vi "Marker Draw and Commands Loop.vi"(9 "Command":T1={"cmd"=enum."type", "Type"=enum."vert", "Coords"={"Horizontal"=0, "Vertical"=0}, "text"=""}, 10 "SPECTRUM":refnum<vi>, 11 "Data in":T7={"PLACEHOLDER"="", "Graph Selection"={"Options"={"Color"=16723218, "pen"={"Width"=2, "Style"=enum."Solid"}, "font"={"Font Name"="Arial", "Size"=14, "Strikeout?"=FALSE, "Italic?"=FALSE, "Underline?"=FALSE, "Outline?"=FALSE, "Shadow?"=FALSE, "Bold?"=FALSE, "FontColor"=6908265}, "caption"="Click to set a point marker"}, "Markers"={"Type"=enum."point", "X"=0.0, "Y"=0.0, "X2"=0.0, "Y2"=0.0, "Text"=""}, "state"={"cmd"=enum."click", "Type"=enum."horiz range", "Coords"={"Horizontal"=0, "Vertical"=0}, "Active Tool"=0, "mode"=enum."none"}}, "Refs"={"Source VI"=refnum, "Graph"=refnum}, "Source Ctrl Label"="", "Channel Peak"=0.0, "Mouse Init Pos"={"Horizontal"=0, "Vertical"=0, "Scrolling"=0}, "Mouse Current Pos"={"Horizontal"=0, "Vertical"=0, "Scrolling"=0}}) -> (3 "Data out":T7={"PLACEHOLDER"="", "Graph Selection"={"Options"={"Color"=16723218, "pen"={"Width"=2, "Style"=enum."Solid"}, "font"={"Font Name"="Arial", "Size"=14, "Strikeout?"=FALSE, "Italic?"=FALSE, "Underline?"=FALSE, "Outline?"=FALSE, "Shadow?"=FALSE, "Bold?"=FALSE, "FontColor"=6908265}, "caption"="Click to set a point marker"}, "Markers"={"Type"=enum."point", "X"=0.0, "Y"=0.0, "X2"=0.0, "Y2"=0.0, "Text"=""}, "state"={"cmd"=enum."click", "Type"=enum."horiz range", "Coords"={"Horizontal"=0, "Vertical"=0}, "Active Tool"=0, "mode"=enum."none"}}, "Refs"={"Source VI"=refnum, "Graph"=refnum}, "Source Ctrl Label"="", "Channel Peak"=0.0, "Mouse Init Pos"={"Horizontal"=0, "Vertical"=0, "Scrolling"=0}, "Mouse Current Pos"={"Horizontal"=0, "Vertical"=0, "Scrolling"=0}})   [LabVIEW 2019]
doc: "This draw loop is the command processor thread and redraw thread to handle the events from the UI. It can be started anywhere with a reference to the graph. Markers work only when the graph palette tool is in cursor mode, as it replaces that mode since Graph extensions have their own improved cursors/markers, that mode is not needed. \n\n<B>Options</B> can be changed by the user using the right click menu with the markers.\n<B>Markers</B> input can be used to initialize a known set of markers (eitehr loaded from disk or programmatically created)\n\n<B>Cursers Enabled</B> activates the other graph extension (cursors) when usual mouse move occurs."
uses:
  controls/Simple Global for Marker Options.vi
  controls/cmd_options.ctl
  controls/MarkerOptions.ctl
  controls/markerType.ctl
  controls/MarkerInfo.ctl
  <vilib>/Utility/miscctls.llb/LVPoint32TypeDef.ctl
  controls/commands.ctl
  controls/GraphExt-Cmds.ctl
panel:
  in  "stop":bool
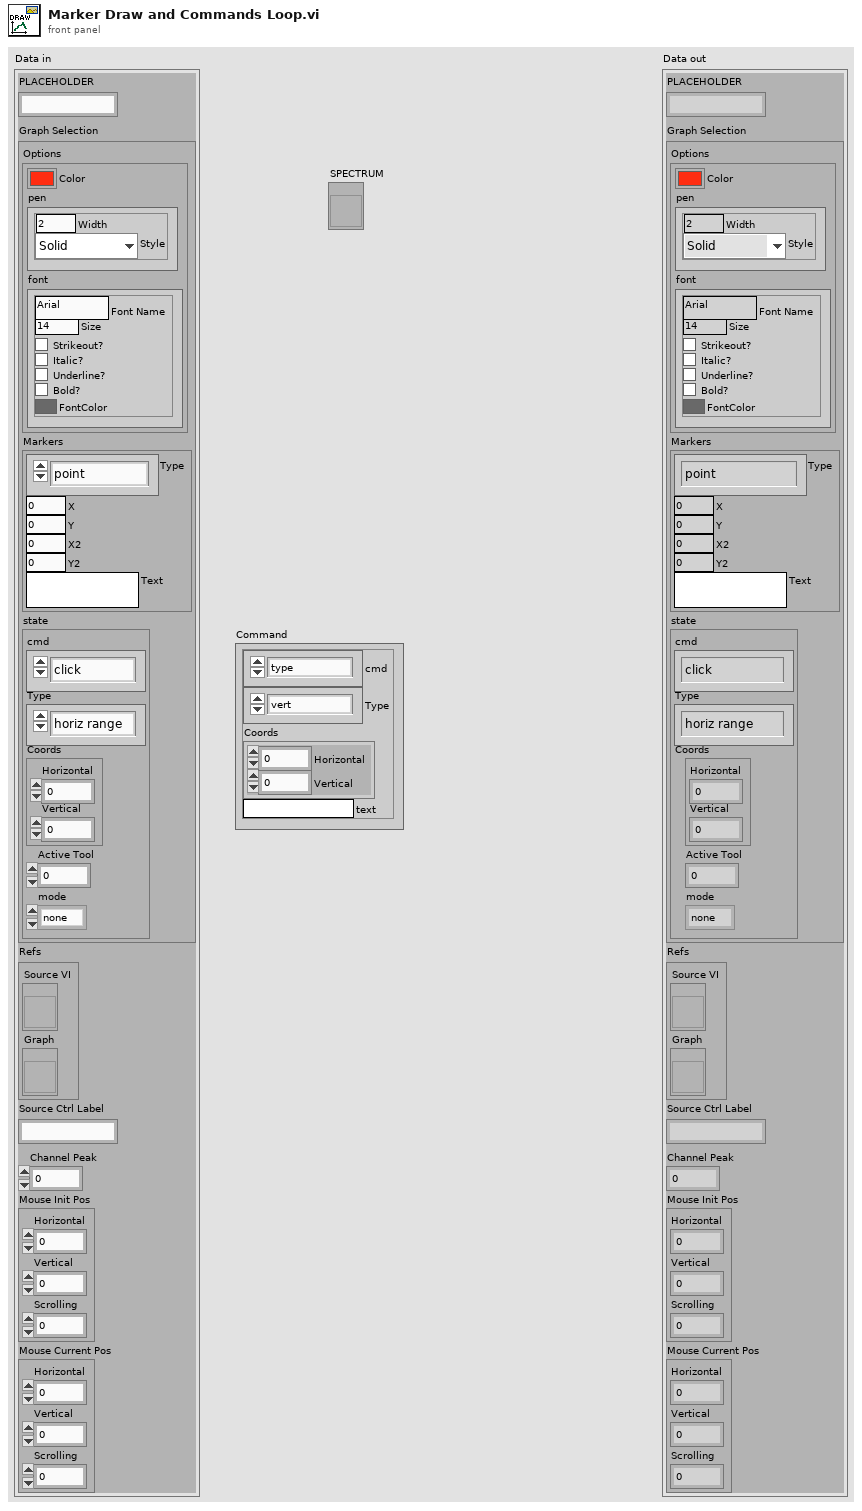
[diagram p1: front panel]
types:
  T1 = typedef "GraphExt-Cmds.ctl" = cluster{"cmd":T2, "Type":T3, "Coords":T4, "text":string}
  T2 = typedef "commands.ctl" = enum16{"up", "options", "click", "move", "type", "redraw", "edited", "exit"}
  T3 = typedef "markerType.ctl" = enum16{"point", "arrow", "horiz", "vert", "vert range", "horiz range", "box"}
  T4 = typedef "LVPoint32TypeDef.ctl" = cluster{"Horizontal":i32, "Vertical":i32}
  T5 = typedef "MarkerOptions.ctl" = cluster{"Color":u32, "pen":cluster{"Width":u16, "Style":enum32{"Solid", "Dash", "Dot", "DashDot", "DashDotDot"}}, "font":cluster{"Font Name":string, "Size":i16, "Strikeout?":bool, "Italic?":bool, "Underline?":bool, "Outline?":bool, "Shadow?":bool, "Bold?":bool, "FontColor":u32}, "caption":string}
  T6 = typedef "MarkerInfo.ctl" = cluster{"Type":T3, "X":dbl, "Y":dbl, "X2":dbl, "Y2":dbl, "Text":string}
  T7 = cluster{"PLACEHOLDER":string, "Graph Selection":cluster{"Options":T5, "Markers":T6, "state":cluster{"cmd":T2, "Type":T3, "Coords":T4, "Active Tool":i32, "mode":enum16{"drag", "none"}}}, "Refs":cluster{"Source VI":refnum<vi>, "Graph":refnum<vi>}, "Source Ctrl Label":string, "Channel Peak":dbl, "Mouse Init Pos":cluster{"Horizontal":i32, "Vertical":i32, "Scrolling":i32}, "Mouse Current Pos":cluster{"Horizontal":i32, "Vertical":i32, "Scrolling":i32}}
  T8 = typedef "cmd_options.ctl" = cluster{"Marker Color":u32, "Style":enum32{"Solid", "Dash", "Dot", "DashDot", "DashDotDot"}, "Width":u16, "Size":i16, "Color":u32}
  T9 = cluster{"cmd":T2, "Type":T3, "Coords":T4, "Active Tool":i32, "mode":enum16{"drag", "none"}}
  T10 = typedef "LVRectTypeDef.ctl" = cluster{"Left":i16, "Top":i16, "Right":i16, "Bottom":i16}
  T11 = enum32{"Solid", "Dash", "Dot", "DashDot", "DashDotDot"}
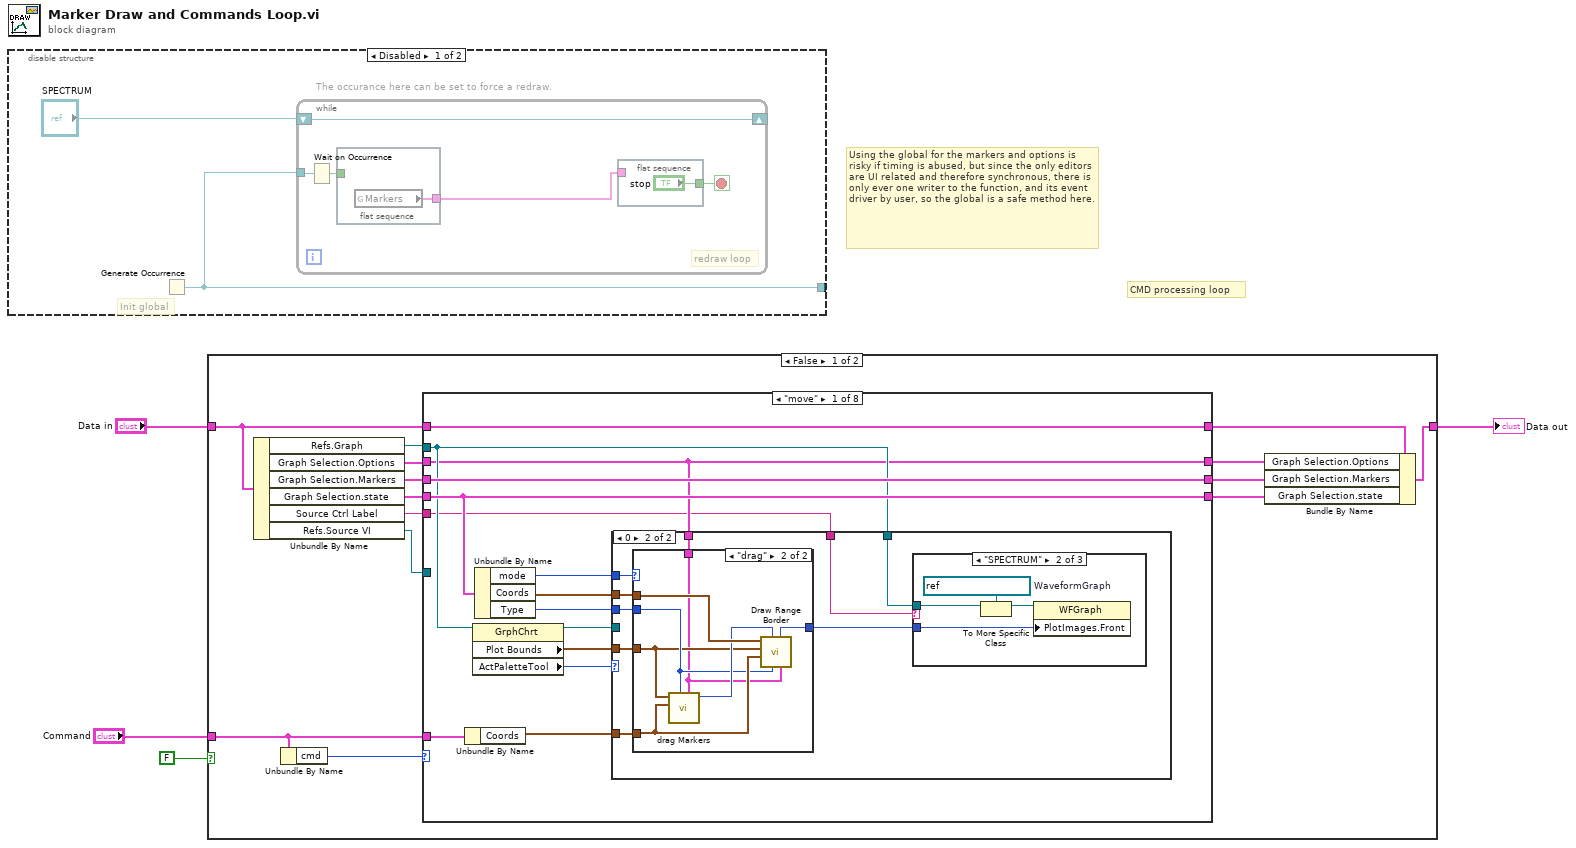
[diagram p0: block diagram]
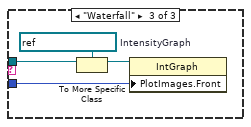
[diagram p4: hidden frame]
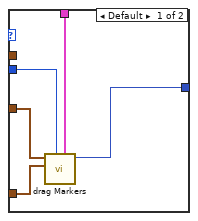
[diagram p5: hidden frame]
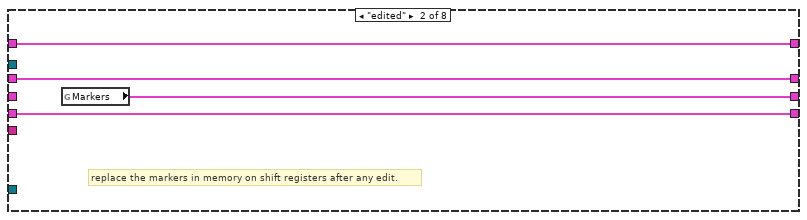
[diagram p6: hidden frame]
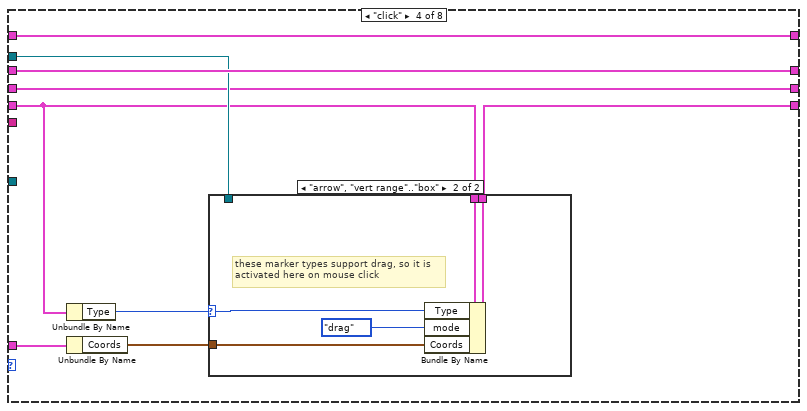
[diagram p8: hidden frame]
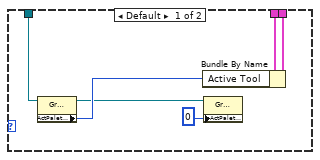
[diagram p9: hidden frame]
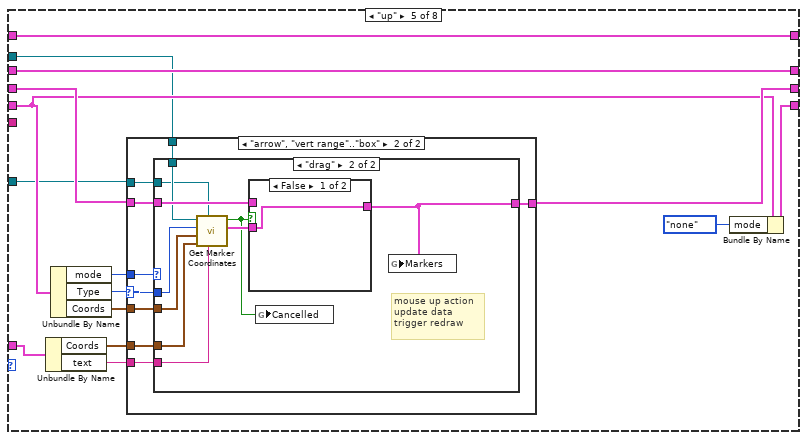
[diagram p10: hidden frame]
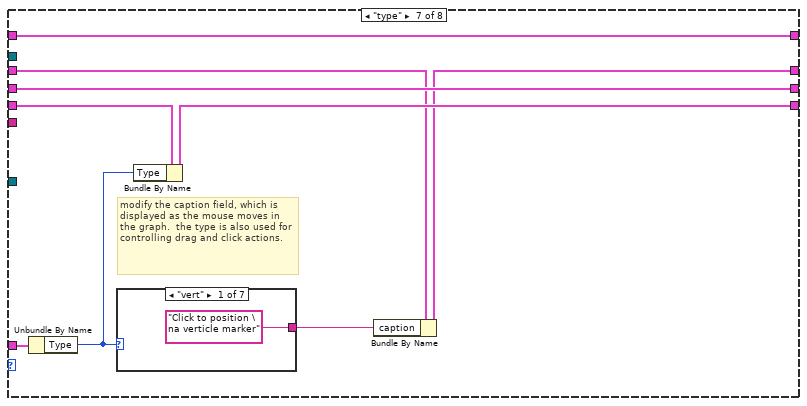
[diagram p15: hidden frame]
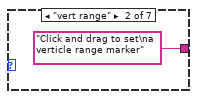
[diagram p16: hidden frame]
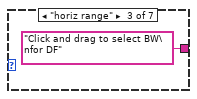
[diagram p17: hidden frame]
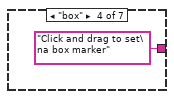
[diagram p18: hidden frame]
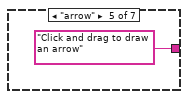
[diagram p19: hidden frame]
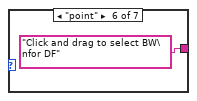
[diagram p20: hidden frame]
diagram:
  # "CMD processing loop"
  # "Using the global for the markers and options is risky if timing is abused, but since the only editors are UI related and therefore synchronous, there is only ever one writer to the function, and its event driver by user, so the global is a safe method here."
  n1 = disable-structure shown="Disabled" {
    disable-tunnel: [w6 _] -> _
    frame Disabled {
      # "Init global"
      # "The occurance here can be set to force a redraw."
      n2 = Generate Occurrence() -> (w6:refnum<k4>)
      n3 = while {
        shift-right: [w7] -> _
        shift-left: "SPECTRUM" -> [w7]
        tunnel: w6 -> [w11]
        stop <- w9 stop-if-true
        # "redraw loop"
        n4 = Wait on Occurrence(2:w11) -> (0:w10:bool)  [unwired: 2 in]
        n5 = flat-sequence {
          tunnel: [w13] -> w8
          tunnel: w10 -> [_]
          frame #0 {
            n6 = global read "Simple Global for Marker Options.vi" "Markers"() -> (w13:T6)
          }
        }
        n7 = flat-sequence {
          tunnel: ["stop"] -> w9
          tunnel: w8 -> [_]
          frame #0 {
          }
        }
      }
    }
    frame Enabled {
    }
  }
  n8 = case shown="False" FALSE ("timed out?") {
    tunnel: "Data in" -> [w27 w171]
    tunnel: [w26 w171] -> w3
    tunnel: "Command" -> [w25 _]
    frame False {
      n9 = Unbundle By Name(w27) -> ("Refs.Graph"=w16:refnum<vi>, "Graph Selection.Options"=w23:T5, "Graph Selection.Markers"=w21:T6, "Graph Selection.state"=w18:T9, "Source Ctrl Label"=w14:string, "Refs.Source VI"=w15:refnum<vi>)
      n10 = Unbundle By Name(w25) -> ("cmd"=w24:T2)
      n11 = case shown="\"move\"" w24 {
        tunnel: w23 -> [w32 w74 w78 w87 w113 w138 w143 w163]
        tunnel: w25 -> [w41 _ _ w86 w112 _ w148 w168]
        tunnel: [w32 w74 w78 w87 w113 w138 w142 w158] -> w20
        tunnel: [w40 w72 w77 w79 w106 w140 w149 w170] -> w19
        tunnel: w21 -> [w40 _ w77 w79 w107 w140 w149 w170]
        tunnel: [w39 w73 w76 w84 w104 w139 w146 w169] -> w17
        tunnel: w18 -> [w39 w73 w76 w83 w105 w139 w147 w169]
        tunnel: w16 -> [w34 _ _ w85 w102 _ _ _]
        tunnel: w27 -> [w29 w71 w75 w80 w101 w137 w141 w157]
        tunnel: [w29 w71 w75 w80 w101 w137 w141 w157] -> w22
        tunnel: w15 -> [_ _ _ _ w99 _ _ _]
        tunnel: w14 -> [w28 _ _ _ _ _ _ _]
        frame "move" {
          n12 = Unbundle By Name(w41) -> ("Coords"=w35:T4)
          n13 = property on="Property Node" class="GrphChrt"(reference=w34) -> (reference out=w30:refnum<vi>, "Plot Bounds"=w33:T10, "ActPaletteTool"=w31:i32)  [unwired: 1 in, 1 out]
          n14 = Unbundle By Name(w39) -> ("mode"=w37:enum16{"drag", "none"}, "Coords"=w38:T4, "Type"=w36:T3)
          n15 = case shown="0" w31 {
            tunnel: w38 -> [_ w50]
            tunnel: w37 -> [_ w48]
            tunnel: w36 -> [_ w47]
            tunnel: w35 -> [_ w46]
            tunnel: w34 -> [_ w45]
            tunnel: w33 -> [_ w44]
            tunnel: w32 -> [_ w43]
            tunnel: w30 -> [_ _]
            tunnel: w28 -> [_ w42]
            frame Default {
              # "ignore markers when not in cursor tool"
            }
            frame 0 {
              n16 = case shown="\"drag\"" w48 {
                tunnel: w50 -> [_ w70]
                tunnel: [w63 w69] -> w49
                tunnel: w43 -> [w62 w64]
                tunnel: w47 -> [w61 w66]
                tunnel: w46 -> [w60 w67]
                tunnel: w44 -> [w59 w65]
                frame Default {
                  n17 = call "drag Markers.vi"("Marker Options"=w62, "Type"=w61, "Coords"=w60, "Plot Area Bounds"=w59) -> ("new picture"=w63:picture)  [unwired: 7 in]
                }
                frame "drag" {
                  n18 = call "drag Markers.vi"("Marker Options"=w64, "Type"=w66, "Coords"=w67, "Plot Area Bounds"=w65) -> ("new picture"=w68:picture)  [unwired: 7 in]
                  n19 = call "Draw Range Border.vi"("Marker Options"=w64, "Type"=w66, "picture"=w68, "end Coords"=w67, "Plot Bounds"=w65, "Start Coords"=w70) -> ("new picture"=w69:picture)  [unwired: 5 in]
                }
              }
              n20 = case shown="\"SPECTRUM\"" w42 {
                tunnel: w49 -> [_ w54 w58]
                tunnel: w45 -> [_ w53 w57]
                frame "False", Default {
                }
                frame "SPECTRUM" {
                  w51 = refnum<vi> refnum  # WaveformGraph
                  n21 = To More Specific Class(target class=w51, reference=w53) -> (specific class reference=w52:refnum<vi>)  [unwired: 1 in, 1 out]
                  n22 = property on="Property Node" class="WFGraph"(reference=w52, "PlotImages.Front"=w54) -> ()  [unwired: 1 in, 2 out]
                }
                frame "Waterfall" {
                  w55 = refnum<vi> refnum  # IntensityGraph
                  n23 = To More Specific Class(target class=w55, reference=w57) -> (specific class reference=w56:refnum<vi>)  [unwired: 1 in, 1 out]
                  n24 = property on="Property Node" class="IntGraph"(reference=w56, "PlotImages.Front"=w58) -> ()  [unwired: 1 in, 2 out]
                }
              }
            }
          }
        }
        frame "edited" {
          # "replace the markers in memory on shift registers after any edit."
          n25 = global read "Simple Global for Marker Options.vi" "Markers"() -> (w72:T6)
        }
        frame "exit" {
        }
        frame "click" {
          n26 = Unbundle By Name(w83) -> ("Type"=w82:T3)
          n27 = Unbundle By Name(w86) -> ("Coords"=w81:T4)
          n28 = case shown="\"arrow\", \"vert range\"..\"box\"" w82 {
            selector: w82 -> [_ w95]
            tunnel: w85 -> [w93 _]
            tunnel: w83 -> [w92 w98]
            tunnel: [w91 w97] -> w84
            tunnel: w81 -> [_ w94]
            frame Default {
              n29 = property class="GrphChrt"(reference=w93) -> (reference out=w89:refnum<vi>, "ActPaletteTool"=w90:i32)  [unwired: 1 in, 1 out]
              n30 = Bundle By Name(cluster=w92, "Active Tool"=w90) -> (w91:T9)
              n31 = property class="GrphChrt"(reference=w89, "ActPaletteTool"=0 ("Palette:Active Tool")) -> ()  [unwired: 1 in, 2 out]
            }
            frame "arrow", "vert range".."box" {
              # "these marker types support drag, so it is\nactivated here on mouse click"
              n32 = Bundle By Name(cluster=w98, "Type"=w95, "mode"=enum16{"drag", "none"}."drag", "Coords"=w94) -> (w97:T9)
            }
          }
        }
        frame "up" {
          n33 = Unbundle By Name(w112) -> ("Coords"=w109:T4, "text"=w100:string)
          n34 = Unbundle By Name(w105) -> ("mode"=w108:enum16{"drag", "none"}, "Type"=w111:T3, "Coords"=w110:T4)
          n35 = case shown="\"arrow\", \"vert range\"..\"box\"" w111 {
            selector: w111 -> [_ w122]
            tunnel: w110 -> [_ w118]
            tunnel: w109 -> [_ w119]
            tunnel: w108 -> [_ w123]
            tunnel: w107 -> [w114 w121]
            tunnel: [w114 w120] -> w106
            tunnel: w102 -> [_ w117]
            tunnel: w100 -> [_ w116]
            tunnel: w99 -> [_ w115]
            frame Default {
              # "mouse up is not supported for these marker types\nor is not needed, since they are single click"
            }
            frame "arrow", "vert range".."box" {
              n36 = case shown="\"drag\"" w123 {
                tunnel: w122 -> [_ w132]
                tunnel: w121 -> [w124 w134]
                tunnel: [w124 w133] -> w120
                tunnel: w119 -> [_ w128]
                tunnel: w118 -> [_ w131]
                tunnel: w117 -> [_ w130]
                tunnel: w116 -> [_ w126]
                tunnel: w115 -> [_ w125]
                frame Default {
                  # "if drag mode was not already active\nthen the up event can be ignored."
                }
                frame "drag" {
                  # "mouse up action\nupdate data\ntrigger redraw"
                  n37 = call "Get Marker Coordinates.vi"("Text"=w126, "Source VI"=w125, "Current Coords"=w128, "Init Coords"=w131, "Type"=w132, "Graph Ref"=w130) -> ("Markers"=w129:T6, "Cancelled"=w127:bool)  [unwired: 4 in]
                  n38 = case shown="False" w127 {
                    tunnel: w134 -> [_ w136]
                    tunnel: [w135 w136] -> w133
                    tunnel: w129 -> [w135 _]
                    frame False {
                    }
                    frame True {
                    }
                  }
                  n39 = global write "Simple Global for Marker Options.vi" "Cancelled"(w127) -> ()
                  n40 = global write "Simple Global for Marker Options.vi" "Markers"(w133) -> ()
                }
              }
            }
          }
          n41 = Bundle By Name(cluster=w105, "mode"=enum16{"drag", "none"}."none") -> (w104:T9)
        }
        frame "redraw" {
        }
        frame "type" {
          # "modify the caption field, which is displayed as the mouse moves in the graph.  the type is also used for controlling drag and click actions."
          n42 = Unbundle By Name(w148) -> ("Type"=w145:T3)
          n43 = case shown="\"vert\"" w145 {
            tunnel: ["Click to position \na verticle marker" ("Text") "Click and drag to set\na verticle range marker" ("Text") "Click and drag to select BW\nfor DF" ("Text") "Click and drag to set\na box marker" ("Text") "Click and drag to draw an arrow" ("Text") "Click and drag to select BW\nfor DF" ("Text") "Click to position \na horizontal marker" ("Text")] -> w144
            frame "vert" {
            }
            frame "vert range" {
            }
            frame "horiz range" {
            }
            frame "box" {
            }
            frame "arrow" {
            }
            frame "point" {
            }
            frame "horiz" {
            }
          }
          n44 = Bundle By Name(cluster=w147, "Type"=w145) -> (w146:T9)
          n45 = Bundle By Name(cluster=w143, "caption"=w144) -> (w142:T5)
        }
        frame "options" {
          # "updates the options for drawing"
          # "Only writer to this global data"
          n46 = Unbundle By Name(w168) -> ("text"=w167:string)
          n47 = Unflatten From String(type=T8 {"Marker Color"=0, "Style"=enum."Solid", "Width"=0, "Size"=0, "Color"=0} ("cluster"), binary string=w167) -> (value=w166:T8)  [unwired: 3 in, 2 out]
          n48 = Unbundle By Name(w166) -> ("Marker Color"=w164:u32, "Style"=w162:T11, "Width"=w161:u16, "Size"=w160:i16, "Color"=w159:u32)
          n49 = Bundle By Name(cluster=w163, "Color"=w164, "pen.Style"=w162, "pen.Width"=w161, "font.Size"=w160, "font.FontColor"=w159) -> (w158:T5)
          n50 = global write "Simple Global for Marker Options.vi" "Options"(w158) -> ()
        }
      }
      n51 = Bundle By Name(cluster=w22, "Graph Selection.Options"=w20, "Graph Selection.Markers"=w19, "Graph Selection.state"=w17) -> (w26:T7)
    }
    frame True {
    }
  }
  "Data out" <- w3
